vi "Test.vi"() -> ()   [LabVIEW 2017]
uses:
  <vilib>/DAQmx/read.llb/DAQmx Read (Analog 1D Wfm NChan NSamp).vi
  <vilib>/DAQmx/miscellaneous.llb/DAQmx Fill In Error Info.vi
panel:
  out "error out":errorcluster
  out "Waveform Graph":waveform(dbl)[](graph)
  in  "DAQmx Task Name":refnum<k21>
  out "Error out (DAQ Loop)":errorcluster
  out "DAQ Loop Iterations":i32
  out "Raw DAQ Output":dynamicdata(graph)=[{"t0"=timestamp(3367839419.335167 s since 1904-01-01), "dt"=0.00016666666666666663, "Y"=array[240 elements], "attributes"=variant("NI_ChannelName"=variant(string "Voltage_0"), "NI_UnitDescription"=variant(string "Volts"))}, {"t0"=timestamp(3367839419.3351874 s since 1904-01-01), "dt"=0.00016666666666666663, "Y"=array[240 elements], "attributes"=variant("NI_ChannelName"=variant(string "Voltage_1"), "NI_UnitDescription"=variant(string "Volts"))}, {"t0"=timestamp(3367839419.3352084 s since 1904-01-01), "dt"=0.00016666666666666663, "Y"=array[240 elements], "attributes"=variant("NI_ChannelName"=variant(string "Voltage_2"), "NI_UnitDescription"=variant(string "Volts"))}]
  in  "All Stop!":bool
  out "Frequency 2":dynamicdata(graph) caption="Frequency"
  out "Phase 2":dynamicdata(graph) caption="Frequency"
  out "Frequency":dbl format="%.2f"
  out "Amplitude":dbl format="%.2f"
  out "Phase":dbl format="%.2f"
  out "Acquisition Time":timestamp
  out "Voltage Waveform":dynamicdata(graph)=[{"t0"=timestamp(3377170241.8512917 s since 1904-01-01), "dt"=0.00016666666666666663, "Y"=array[300 elements]}, {"t0"=timestamp(3377170241.8513126 s since 1904-01-01), "dt"=0.00016666666666666663, "Y"=array[300 elements]}, {"t0"=timestamp(3377170241.8513336 s since 1904-01-01), "dt"=0.00016666666666666663, "Y"=array[300 elements]}]
  out "IP":string
  out "Port":i32
  out "Transmitted Data":string
  out "Stop":bool
  out "Elements in Acquisition Buffer":i32
  # "V1.2 - PFI0 (Single Phase)"
  # "50.5"
  # "The code and design of this VI are licensed \nunder the terms of the New BSD License.\nPlease see the VI documentation or License.txt\nfor more details.\n\nCopyright (c) 2012, David Laverty\nwww.OpenPMU.org"
  # "Configuration Information:\n\nThe ID and IP address to which the OpenPMU sends data is configured by 'C:\\PMUconfig.ini'.  If this doesn't exist, create it.\n\nCopy and paste the blue text below without the dashed lines into PMUconfig.ini.\n\n[Telecoms]\nID=PMU123\nIP=192.168.1.100\nPort=40001\n\nIP and Port may be any values within normal IPv4 range.  ID should be six alpha-numeric characters."
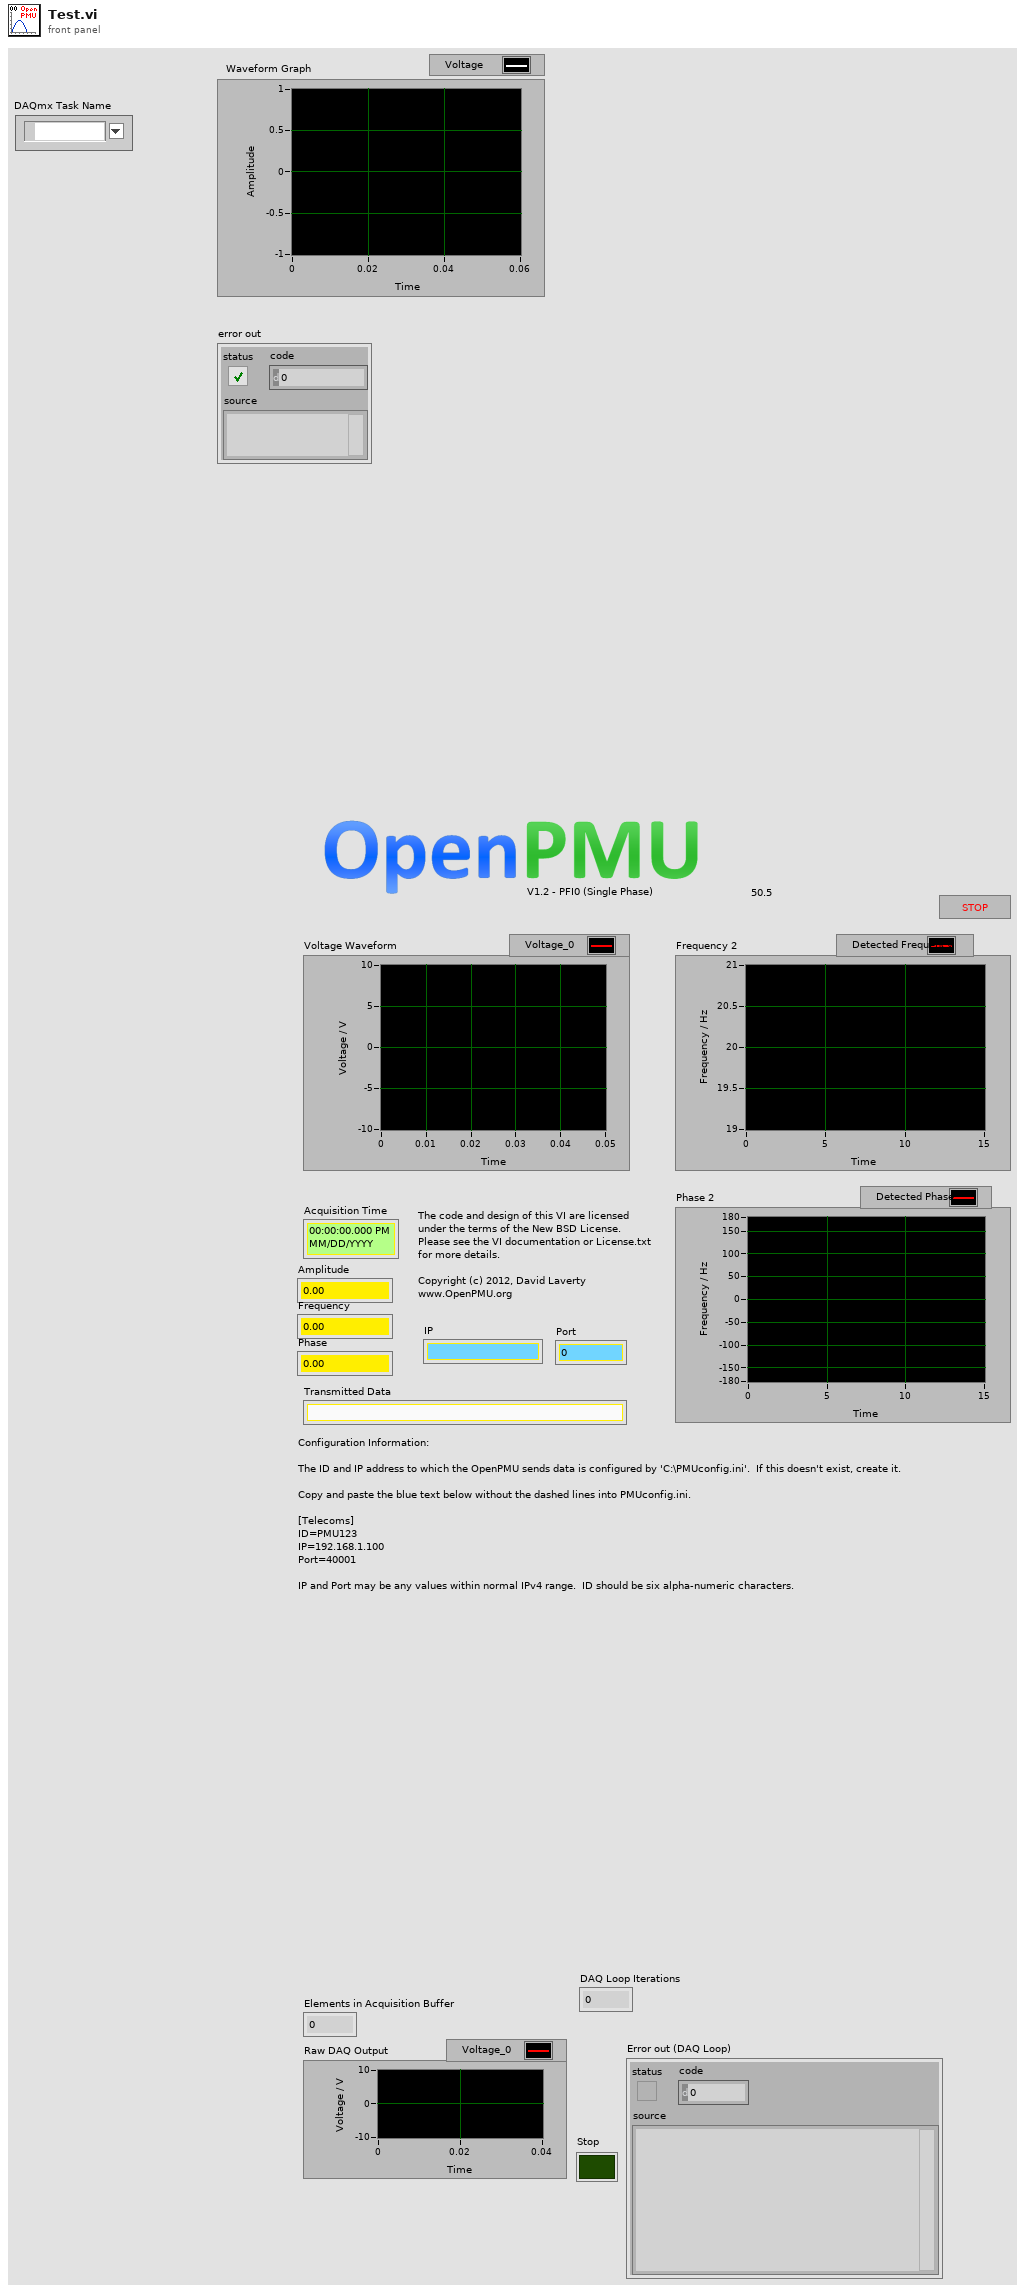
[diagram p1: front panel]
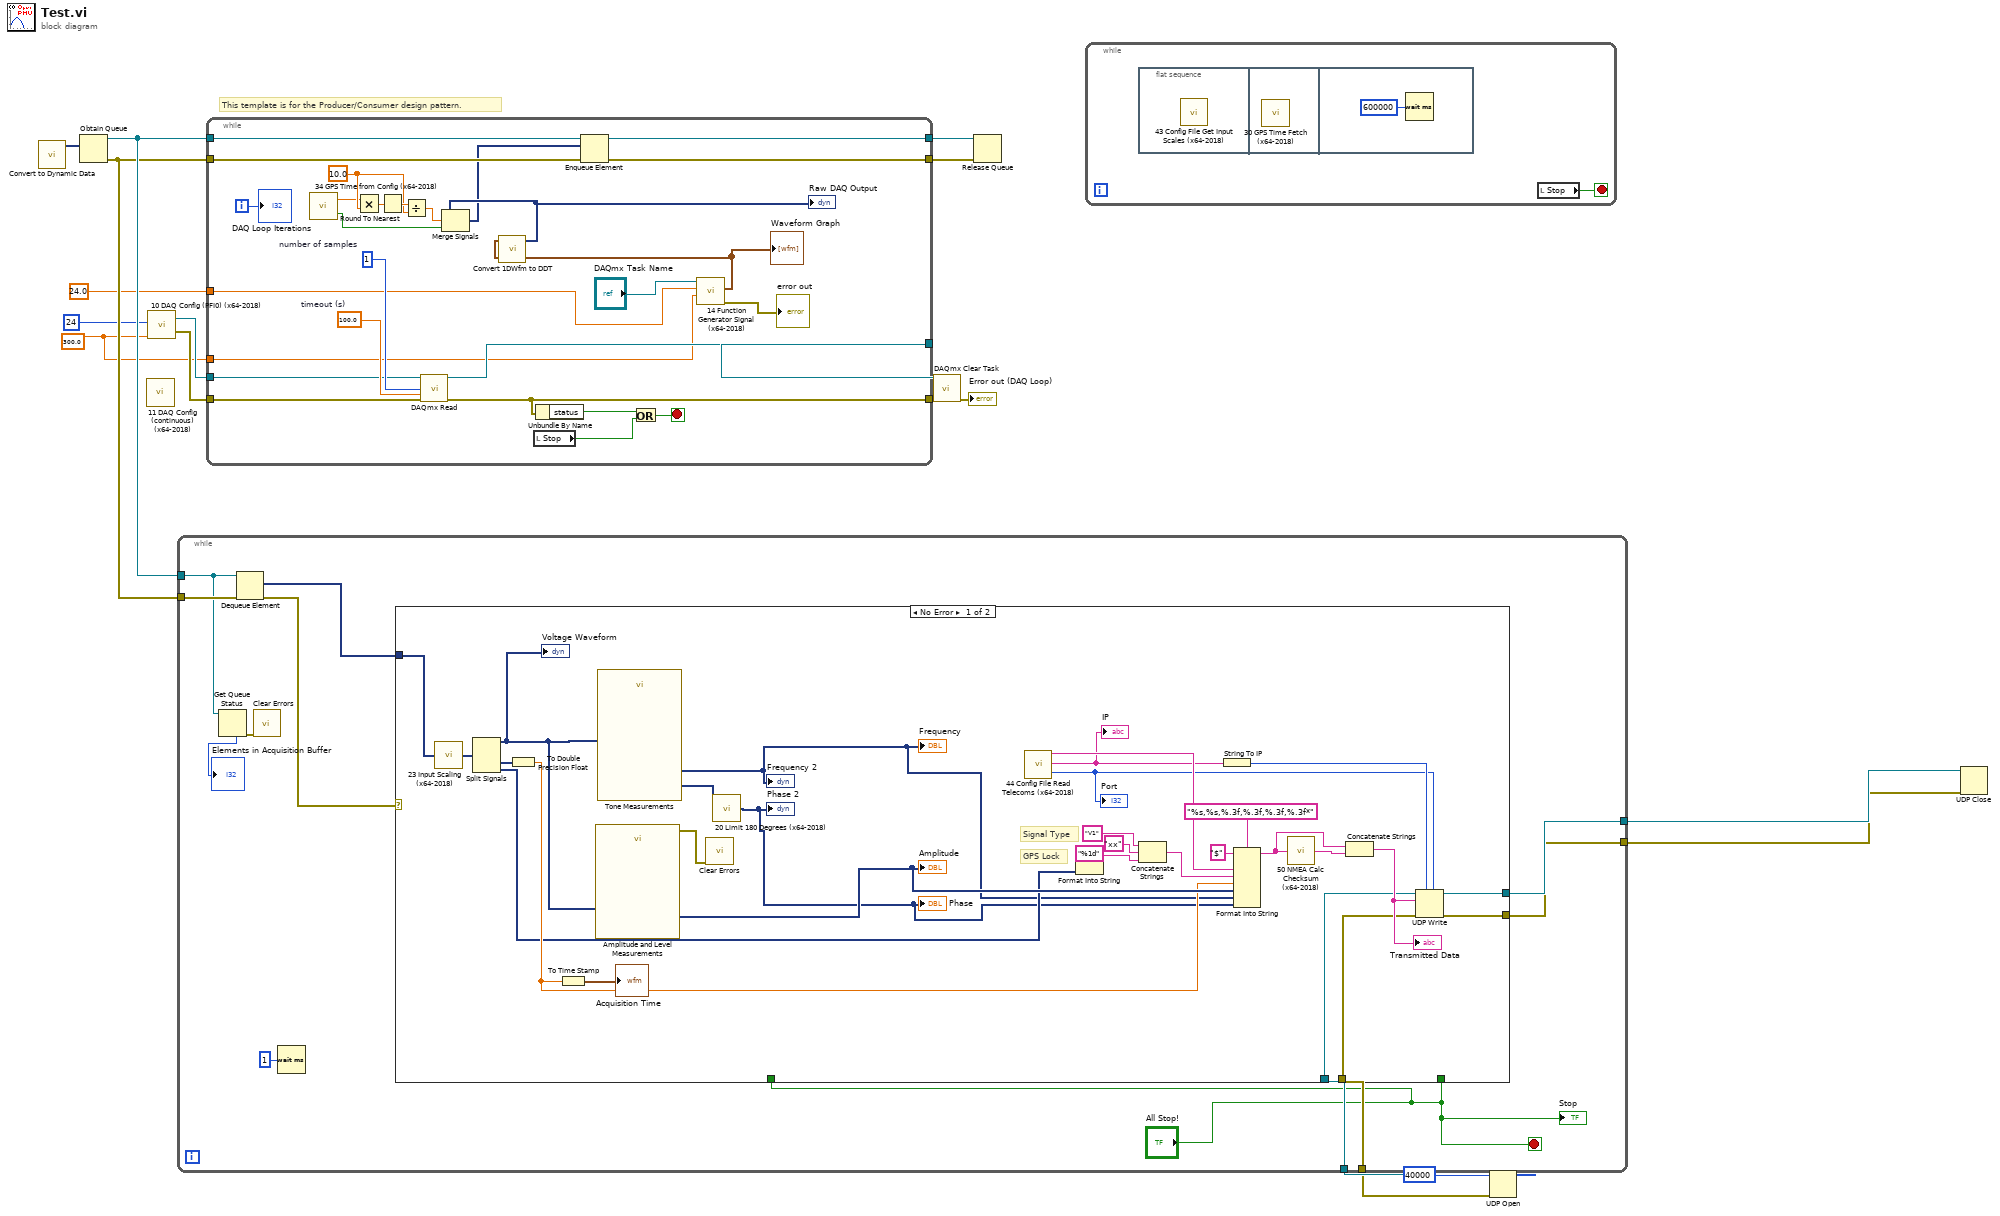
[diagram p0: block diagram]
diagram:
  w1 = 300.0 ("rate")
  # "This template is for the Producer/Consumer design pattern."
  n1 = call "Convert to Dynamic Data"() -> ("Dynamic Data Type"=w15:dynamicdata)  [unwired: 4 in]
  n2 = Obtain Queue(element data type=w15) -> (queue out=w12:refnum<queue>, error out=w11:errorcluster)  [unwired: 4 in, 1 out]
  n3 = call "11 DAQ Config (continuous) (x64-2018).vi"() -> ()  [unwired: 1 in, 2 out]
  n4 = call "10 DAQ Config (PFI0) (x64-2018).vi"("rate"=w1, "number of samples"=24) -> ("Error Out"=w4:errorcluster, "task out"=w5:refnum<k21>)  [unwired: 1 in]
  n5 = while {
    tunnel: w4 -> [w32]
    tunnel: w5 -> [w33]
    tunnel: [w42] -> w18
    tunnel: [w41] -> w17
    tunnel: w12 -> [w37]
    tunnel: w11 -> [w36]
    tunnel: [w35] -> w14
    tunnel: [w34] -> w13
    tunnel: 24.0 -> [w21]
    tunnel: w1 -> [w20]
    i -> [w40]
    stop <- w39 stop-if-true
    w26 = 10.0 ("y")
    w43 = 100.0  # timeout (s)
    w45 = 1  # number of samples
    n6 = call "34 GPS Time from Config (x64-2018).vi"() -> ("GPS Lock"=w24:bool, "Time"=w25:dbl)  [unwired: 2 in]
    n7 = Multiply(x=w25, y=w26) -> (x*y=w29:dbl)
    n8 = Round To Nearest(number=w29) -> (nearest integer value=w28:dbl)
    n9 = Divide(x=w28, y=w26) -> (x/y=w27:dbl)
    n10 = call-poly <vilib>:"DAQmx Read.vi"("task/channels in"=w33, "number of samples per channel"=w45, "timeout"=w43, "error in"=w32) -> ("task out"=w42:refnum<k21>, "error out"=w41:errorcluster)  [unwired: 9 in, 1 out]
    n11 = local read "Stop"() -> (w38:bool)
    n12 = Unbundle By Name(w41) -> ("status"=w44:bool)
    n13 = Or(x=w44, y=w38) -> (x .or. y?=w39:bool)
    n14 = call "14 Function Generator Signal (x64-2018).vi"("Rate"=w20, "Number of samples per channel"=w21, "task/channels in"="DAQmx Task Name") -> ("Error Out"=→"error out":errorcluster, "data"=w19:waveform(dbl)[])  [unwired: 6 in, 1 out]
    "Waveform Graph" <- w19
    n15 = call <vilib>:"Convert 1DWfm to DDT.vi"("Array of Waveforms"=w19) -> ("Dynamic Data Type"=w31:dynamicdata)  [unwired: 3 in]
    "Raw DAQ Output" <- w31
    n16 = Merge Signals(w31, w27, w24) -> (w30:dynamicdata)
    n17 = Enqueue Element(queue=w37, element=w30, error in (no error)=w36) -> (queue out=w35:refnum<queue>, error out=w34:errorcluster)  [unwired: 1 in, 1 out]
    "DAQ Loop Iterations" <- w40
  }
  n18 = call <vilib>:"DAQmx Clear Task.vi"("task in"=w18, "error in"=w17) -> ("error out"=→"Error out (DAQ Loop)":errorcluster)  [unwired: 13 in]
  n19 = Release Queue(queue=w14, error in (no error)=w13) -> ()  [unwired: 1 in, 3 out]
  n20 = while {
    stop <- w46 stop-if-true
    n21 = flat-sequence {
      frame #0 {
        n22 = call "43 Config File Get Input Scales (x64-2018).vi"() -> ()  [unwired: 1 in]
      }
      frame #1 {
        n23 = call "30 GPS Time Fetch (x64-2018).vi"() -> ()  [unwired: 1 in]
      }
      frame #2 {
        n24 = Wait (ms)(milliseconds to wait=u32 600000) -> ()  [unwired: 1 out]
      }
    }
    n25 = local read "Stop"() -> (w46:bool)
  }
  n26 = UDP Open(11:u16 40000 ("port")) -> (port=w9:refnum<k16>, 0:w8:errorcluster)  [unwired: 4 in, 1 out]
  n27 = while {
    tunnel: w12 -> [w54]
    tunnel: w11 -> [w56]
    tunnel: w9 -> [w53]
    tunnel: w8 -> [w52]
    tunnel: [w51] -> w7
    tunnel: [w50] -> w6
    stop <- "All Stop!" stop-if-true
    n28 = Get Queue Status(queue=w54) -> (error out=w49:errorcluster, # elements in queue=→"Elements in Acquisition Buffer":i32)  [unwired: 2 in, 6 out]
    n29 = Dequeue Element(queue=w54, error in (no error)=w56) -> (element=w57:dynamicdata, error out=w58:errorcluster)  [unwired: 1 in, 2 out]
    n30 = call <vilib>:"Clear Errors.vi"("error in (no error)"=w49) -> ()  [unwired: 5 in, 2 out]
    n31 = Wait (ms)(milliseconds to wait=u32 1) -> ()  [unwired: 1 out]
    n32 = case shown="No Error" w58 {
      tunnel: w57 -> [w70 _]
      tunnel: w53 -> [w83 w91]
      tunnel: w52 -> [w82 w90]
      tunnel: [w81 w91] -> w51
      tunnel: [w80 w90] -> w50
      tunnel: "All Stop!" -> [_ _]
      tunnel: "All Stop!" -> [_ _]
      frame No Error {
        # "GPS Lock"
        # "Signal Type"
        n33 = call "23 Input Scaling (x64-2018).vi"("Input (Raw)"=w70) -> ("Output (Scaled)"=w69:dynamicdata)
        n34 = Split Signals(w69) -> (w60:dynamicdata, w79:dynamicdata, w76:dynamicdata)  [unwired: 5 in, 2 out]
        "Voltage Waveform" <- w60
        n35 = To Double Precision Float(number=w79) -> (double precision float=w77:dbl)
        n36 = To Time Stamp(1:w77) -> (0:→"Acquisition Time":timestamp)
        n37 = call "Amplitude and Level Measurements"("Signals"=w60) -> ("Cycle RMS"=w78:dynamicdata, "error out"=w89:errorcluster)  [unwired: 13 in]
        "Amplitude" <- w78
        n38 = call "Tone Measurements"("Signals"=w60) -> ("Phase"=w68:dynamicdata, "Frequency"=w62:dynamicdata)  [unwired: 7 in, 2 out]
        "Frequency 2" <- w62
        "Frequency" <- w62
        n39 = call <vilib>:"Clear Errors.vi"("error in (no error)"=w89) -> ()  [unwired: 5 in, 2 out]
        n40 = call "20 Limit 180 Degrees (x64-2018).vi"("Angle In"=w68) -> ("Angle Out"=w61:dynamicdata)
        "Phase 2" <- w61
        "Phase" <- w61
        n41 = call "44 Config File Read Telecoms (x64-2018).vi"() -> ("Port"=w65:i32, "IP"=w66:string, "ID"=w67:string)  [unwired: 3 in]
        "IP" <- w66
        "Port" <- w65
        n42 = Format Into String(format string="%1d", w76) -> (resulting string=w71:string)  [unwired: 2 in, 1 out]
        n43 = Concatenate Strings("V1" ("input 2"), "xx" ("string"), w71) -> (w73:string)
        n44 = String To IP(1:w66) -> (0:w85:u32)
        n45 = Format Into String(format string="%s,%s,%.3f,%.3f,%.3f,%.3f*", initial string="$", w67, w73, w77, w78, w62, w61) -> (resulting string=w64:string)  [unwired: 1 in, 1 out]
        n46 = call "50 NMEA Calc Checksum (x64-2018).vi"("GPS String"=w64) -> ("hex integer string"=w63:string)  [unwired: 1 in, 1 out]
        n47 = Concatenate Strings(w64, w63) -> (w84:string)
        "Transmitted Data" <- w84
        n48 = UDP Write(address=w85, port or service name=w65, connection ID=w83, data in=w84, 8:w82) -> (error out=w80:errorcluster, 3:w81:refnum<k16>)  [unwired: 1 in]
      }
      frame Error {
      }
    }
    "Stop" <- "All Stop!"
  }
  n49 = UDP Close(connection ID=w7, 8:w6) -> ()  [unwired: 2 out]
